vi "Dual_DM_Control_Main_V6.vi"() -> ()   [LabVIEW 2014]
uses:
  Controls/MirrorModes.ctl
  Controls/Standard Action.ctl
  <vilib>/Analysis/baseanly.llb/Mean (DBL).vi
  <vilib>/Utility/file.llb/Write To Spreadsheet File (DBL).vi
  <vilib>/Utility/file.llb/Read From Spreadsheet File (DBL).vi
  <vilib>/Analysis/NI_AALBase.lvlib
panel:
  out "Pixel Map (-1 to 1) 2":dbl[][](graph)
  in  "Python":bool
  in  "Control Mode":T1(radio)
  in  "Active Mirror":enum32{"Mirror 1", "Mirror 2"}(radio)
  in  "Clear Modes":bool
  in  "Mirror Modes":T2
  in  "Load Modes":bool
  in  "Save Modes":bool
  in  "Scan Modes":bool
  in  "Load Flat":bool
  in  "Apply Zero":bool
  in  "Load V Map":bool
  in  "Save V Map":bool
  in  "Apply Flat":bool=TRUE
  in  "Center Bias":bool
  in  "Exit":bool
  out "Pixel Map (-1 to 1)":dbl[][](graph)
  # "Mode"
  # "Amount (nm)"
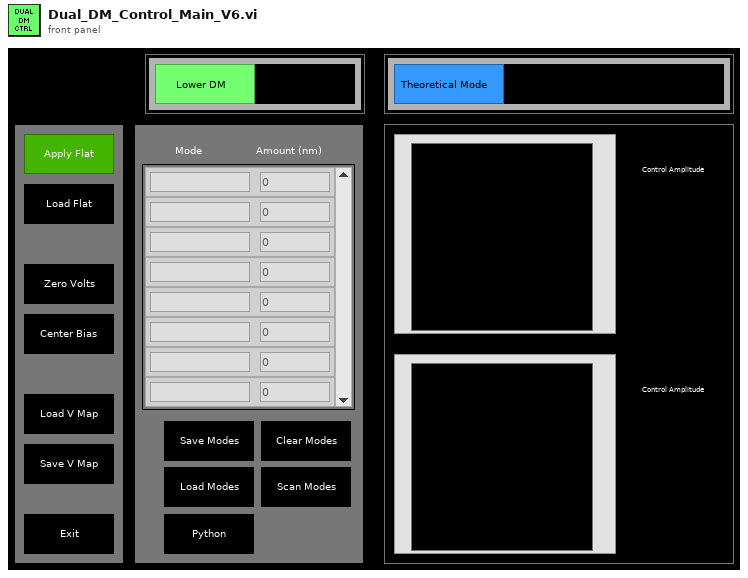
[diagram p1: front panel]
types:
  T1 = enum32{"Theoretical Mode", "Practical Mode", "Poke"}
  T2 = typedef "MirrorModes.ctl" = cluster{"Mode":string, "Amplitude":dbl}[]
  T3 = typedef "Standard Action.ctl" = enum16{"Read", "Write"}
  T4 = typedef "MirrorModes_DUAL.ctl" = cluster{"Mode":string, "Amplitude":dbl}[][]
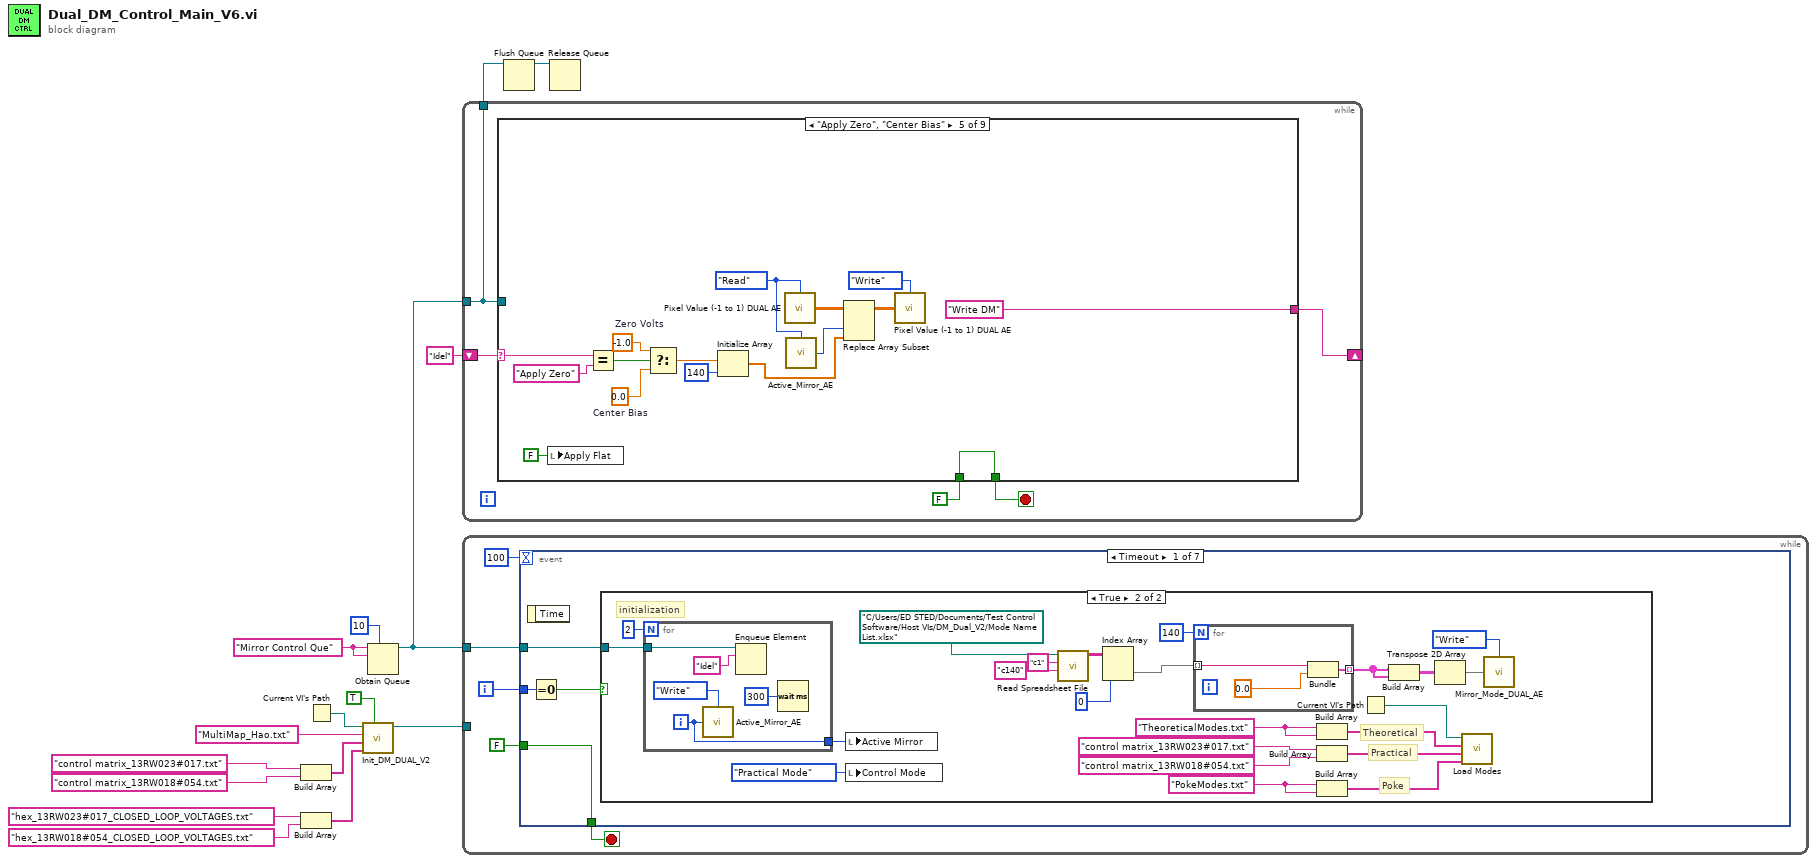
[diagram p0: block diagram]
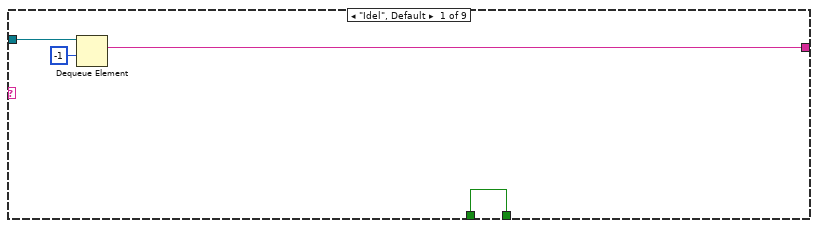
[diagram p2: hidden frame]
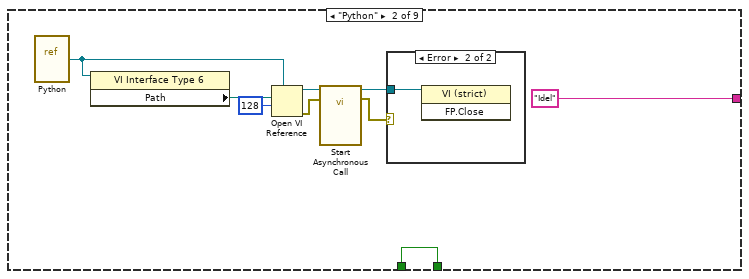
[diagram p3: hidden frame]
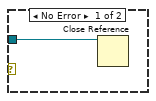
[diagram p4: hidden frame]
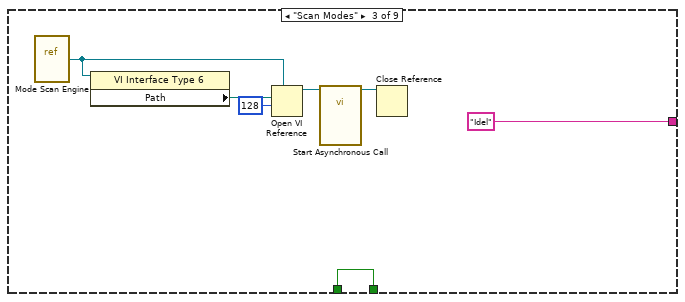
[diagram p5: hidden frame]
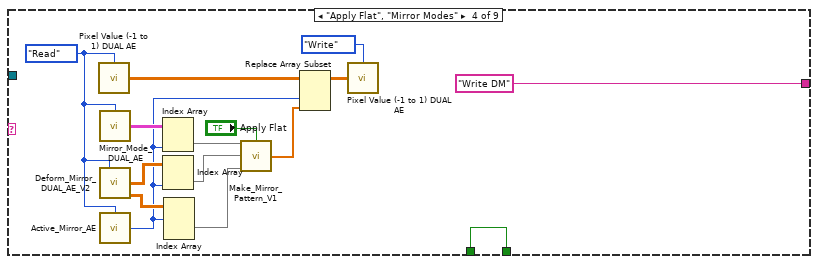
[diagram p6: hidden frame]
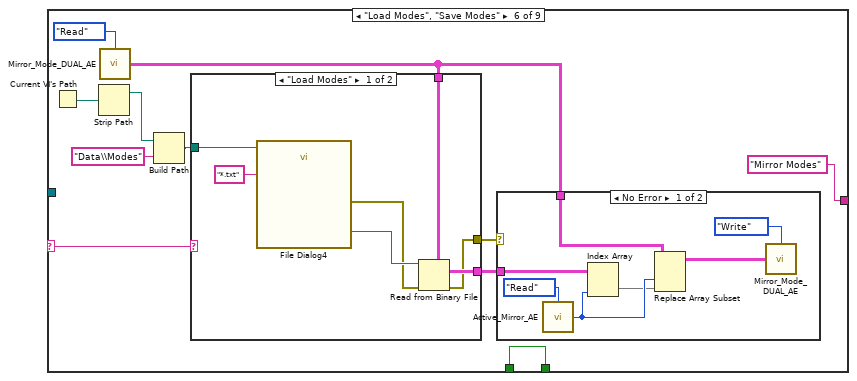
[diagram p7: hidden frame]
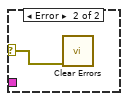
[diagram p8: hidden frame]
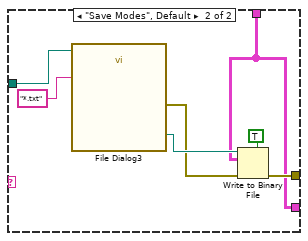
[diagram p9: hidden frame]
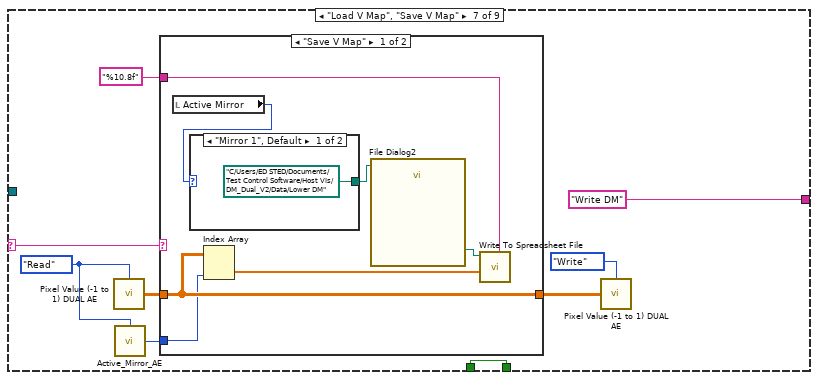
[diagram p10: hidden frame]
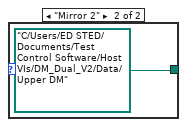
[diagram p11: hidden frame]
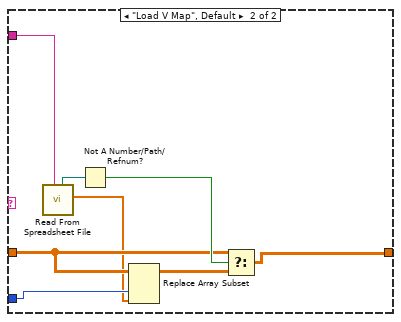
[diagram p12: hidden frame]
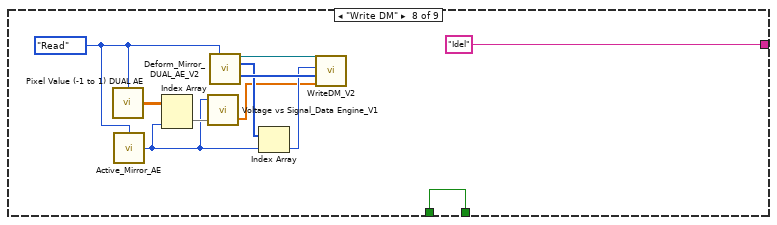
[diagram p13: hidden frame]
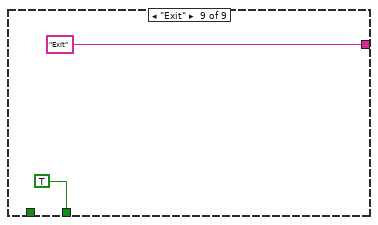
[diagram p14: hidden frame]
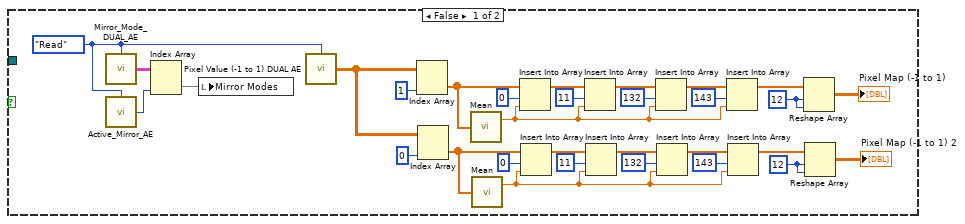
[diagram p15: hidden frame]
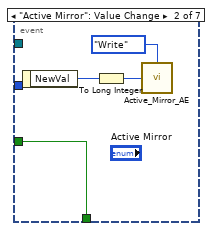
[diagram p16: hidden frame]
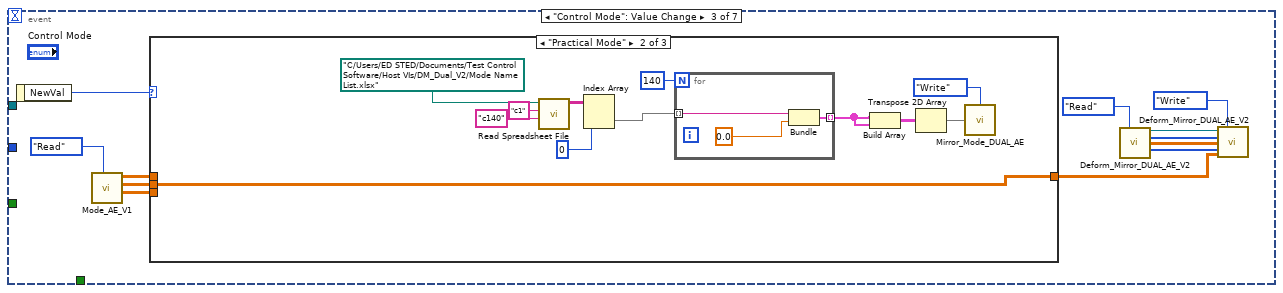
[diagram p17: hidden frame]
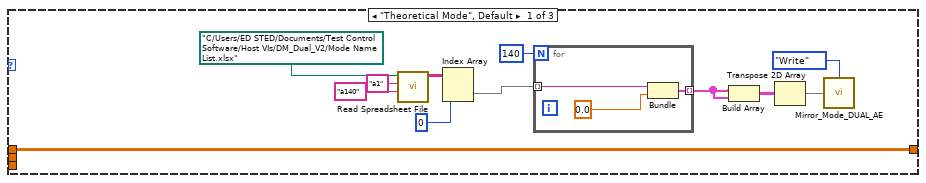
[diagram p18: hidden frame]
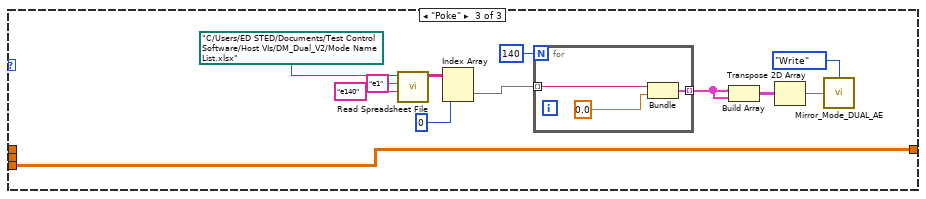
[diagram p19: hidden frame]
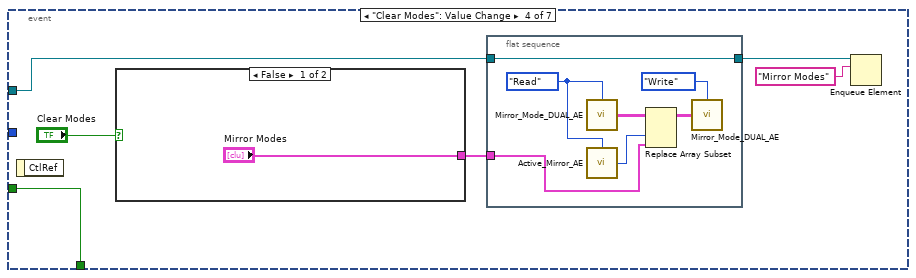
[diagram p20: hidden frame]
diagram:
  w16 = "Mirror Control Que" ("name (unnamed)")
  n1 = Build Array("control matrix_13RW023#017.txt" ("name or relative path"), "control matrix_13RW018#054.txt" ("name or relative path")) -> (w3:string[])
  n2 = Build Array("hex_13RW023#017_CLOSED_LOOP_VOLTAGES.txt" ("name or relative path"), "hex_13RW018#054_CLOSED_LOOP_VOLTAGES.txt" ("name or relative path")) -> (w6:string[])
  n3 = Current VI's Path() -> (path=w8:path)
  n4 = call "Init_DM_DUAL_V2.vi"("BM Flat"=TRUE, "BM Flat File"=w6, "Control Mode In"=w3, "DM Mapping File"="MultiMap_Hao.txt" ("name or relative path"), "Base File Path"=w8) -> ("reference out"=w14:refnum<k7>)  [unwired: 6 in]
  n5 = Obtain Queue(max queue size (-1, unlimited)=10, name (unnamed)=w16, element data type=w16) -> (queue out=w10:refnum<queue>)  [unwired: 2 in, 2 out]
  n6 = while {
    tunnel: w10 -> [w17]
    shift-right: [w21] -> _
    shift-left: "Idel" ("name (unnamed)") -> [w20]
    tunnel: [w17] -> w13
    stop <- w19 stop-if-true
    n7 = case shown="\"Apply Zero\", \"Center Bias\"" w20 {
      selector: w20 -> [_ _ _ _ w70 w82 w115 _ _]
      tunnel: w17 -> [w25 _ _ _ _ _ _ _ _]
      tunnel: [w23 "Idel" ("name (unnamed)") "Idel" ("name (unnamed)") "Write DM" ("name (unnamed)") "Write DM" ("name (unnamed)") "Mirror Modes" ("name (unnamed)") "Write DM" ("name (unnamed)") "Idel" ("name (unnamed)") "Exit" ("name (unnamed)")] -> w21
      tunnel: [w22 w28 w42 w57 w74 w85 w116 w144 TRUE] -> w19
      tunnel: FALSE -> [w22 w28 w42 w57 w74 w85 w116 w144 _]
      frame "Idel", Default {
        n8 = Dequeue Element(queue=w25, timeout in ms (-1)=-1) -> (element=w23:string)  [unwired: 1 in, 3 out]
      }
      frame "Python" {
        n9 = vi-ref "Python.vi"() -> (w29:refnum<vi>)
        n10 = property class="VI Interface Type 6"(reference=w29) -> ("Path"=w30:path)  [unwired: 1 in, 2 out]
        n11 = Open VI Reference(type specifier VI Refnum (for type only)=w29, vi path=w30, options=128) -> (vi reference=w32:refnum<vi>, error out=w27:errorcluster)  [unwired: 3 in]
        n12 = call-by-ref "Start Asynchronous Call"(reference=w32, error in=w27) -> (reference out=w33:refnum<vi>, error out=w26:errorcluster)  [unwired: 2 in]
        n13 = case shown="Error" w26 {
          tunnel: w33 -> [w35 w36]
          frame No Error {
            n14 = Close Reference(reference=w35) -> ()  [unwired: 1 in, 1 out]
          }
          frame Error {
            n15 = invoke class="VI (strict)" method="FP.Close"(reference=w36) -> ()  [unwired: 2 in, 3 out]
          }
        }
      }
      frame "Scan Modes" {
        n16 = vi-ref "Mode Scan Engine.vi"() -> (w37:refnum<vi>)
        n17 = property class="VI Interface Type 6"(reference=w37) -> ("Path"=w38:path)  [unwired: 1 in, 2 out]
        n18 = Open VI Reference(type specifier VI Refnum (for type only)=w37, vi path=w38, options=128) -> (vi reference=w40:refnum<vi>)  [unwired: 3 in, 1 out]
        n19 = call-by-ref "Start Asynchronous Call"(reference=w40) -> (reference out=w41:refnum<vi>)  [unwired: 3 in, 1 out]
        n20 = Close Reference(reference=w41) -> ()  [unwired: 1 in, 1 out]
      }
      frame "Apply Flat", "Mirror Modes" {
        w53 = Standard_Action."Read" ("Action")
        n21 = call "Pixel Value (-1 to 1) DUAL AE.vi"("Action"=w53) -> ("Pixel Value (-1 to 1) Out"=w54:dbl[][])  [unwired: 14 in]
        n22 = call "Mirror_Mode_DUAL_AE.vi"("Action"=w53) -> ("Mirror Modes Out"=w50:T4)  [unwired: 14 in]
        n23 = call "Deform_Mirror_DUAL_AE_V2.vi"("Action"=w53) -> ("Flat Files Out"=w48:dbl[][], "Mode Matrix Out"=w46:dbl[][][])  [unwired: 10 in, 3 out]
        n24 = call "Active_Mirror_AE.vi"("Action"=w53) -> ("Active Mirror"=w44:i32)  [unwired: 14 in]
        n25 = Index Array(array=w50, index (col)=w44) -> (element=w51:cluster{"Mode":string, "Amplitude":dbl}[])  [unwired: 1 in]
        n26 = Index Array(array=w48, index (col)=w44) -> (element=w49:dbl[])  [unwired: 1 in]
        n27 = Index Array(array=w46, index (dim 0)=w44) -> (element=w45:dbl[][])  [unwired: 2 in]
        n28 = call "Make_Mirror_Pattern_V1.vi"("Mirror Modes In"=w51, "Flat On?"="Apply Flat", "Flat File In"=w49, "Mirror Modes Array"=w45) -> ("Pixel Value U (-1 to 1)"=w55:dbl[])  [unwired: 11 in]
        n29 = Replace Array Subset(array=w54, new element=w55, index (col)=w44) -> (w56:dbl[][])  [unwired: 1 in]
        n30 = call "Pixel Value (-1 to 1) DUAL AE.vi"("Action"=Standard_Action."Write", "Pixel Value (-1 to 1)"=w56) -> ()  [unwired: 13 in, 1 out]
      }
      frame "Apply Zero", "Center Bias" {
        w63 = Standard_Action."Read" ("Action")
        w66 = -1.0  # Zero Volts
        w68 = 0.0  # Center Bias
        n31 = local write "Apply Flat"(FALSE ("Apply Flat")) -> ()
        n32 = Equal?(x=w70, y="Apply Zero") -> (x = y?=w69:bool)
        n33 = Select(t=w66, s=w69, f=w68) -> (s? t:f=w67:dbl)
        n34 = Initialize Array(w67, 140 ("dimension size")) -> (w60:dbl[])
        n35 = call "Pixel Value (-1 to 1) DUAL AE.vi"("Action"=w63) -> ("Pixel Value (-1 to 1) Out"=w61:dbl[][])  [unwired: 14 in]
        n36 = call "Active_Mirror_AE.vi"("Action"=w63) -> ("Active Mirror"=w62:i32)  [unwired: 14 in]
        n37 = Replace Array Subset(array=w61, new element=w60, index (col)=w62) -> (w64:dbl[][])  [unwired: 1 in]
        n38 = call "Pixel Value (-1 to 1) DUAL AE.vi"("Action"=Standard_Action."Write", "Pixel Value (-1 to 1)"=w64) -> ()  [unwired: 13 in, 1 out]
      }
      frame "Load Modes", "Save Modes" {
        n39 = Current VI's Path() -> (path=w80:path)
        n40 = Strip Path(path=w80) -> (stripped path=w79:path)  [unwired: 1 out]
        n41 = call "Mirror_Mode_DUAL_AE.vi"("Action"=Standard_Action."Read") -> ("Mirror Modes Out"=w75:T4)  [unwired: 14 in]
        n42 = Build Path(base path=w79, name or relative path="Data\\Modes") -> (appended path=w77:path)
        n43 = case shown="\"Load Modes\"" w82 {
          tunnel: w75 -> [w94 w101]
          tunnel: [w100 w101] -> w81
          tunnel: w77 -> [w99 w106]
          tunnel: [w96 w103] -> w76
          frame "Load Modes" {
            n44 = call "File Dialog4"("start path"=w99, "pattern (all files)"="*.txt") -> ("selected path"=w98:path, "error out"=w95:errorcluster)  [unwired: 10 in, 2 out]
            n45 = Read from Binary File(5:w94, 8:w95, 11:w98) -> (0:w96:errorcluster, 2:w100:T4)  [unwired: 3 in, 2 out]
          }
          frame "Save Modes", Default {
            n46 = call "File Dialog3"("start path"=w106, "pattern (all files)"="*.txt") -> ("selected path"=w105:path, "error out"=w102:errorcluster)  [unwired: 10 in, 2 out]
            n47 = Write to Binary File(file (use dialog)=w105, data=w101, error in=w102, 5:TRUE ("prepend array or string size? (T)")) -> (error out=w103:errorcluster)  [unwired: 2 in, 2 out]
          }
        }
        n48 = case shown="No Error" w76 {
          selector: w76 -> [_ w93]
          tunnel: w81 -> [w91 _]
          tunnel: w75 -> [w89 _]
          frame No Error {
            n49 = call "Active_Mirror_AE.vi"("Action"=Standard_Action."Read") -> ("Active Mirror"=w88:i32)  [unwired: 14 in]
            n50 = Index Array(array=w91, index (col)=w88) -> (element=w87:cluster{"Mode":string, "Amplitude":dbl}[])  [unwired: 1 in]
            n51 = Replace Array Subset(array=w89, new element=w87, index (col)=w88) -> (w86:T4)  [unwired: 1 in]
            n52 = call "Mirror_Mode_DUAL_AE.vi"("Action"=Standard_Action."Write", "Mirror Modes In"=w86) -> ()  [unwired: 13 in, 1 out]
          }
          frame Error {
            n53 = call <vilib>:"Clear Errors.vi"("error in (no error)"=w93) -> ()  [unwired: 5 in, 2 out]
          }
        }
      }
      frame "Load V Map", "Save V Map" {
        w109 = Standard_Action."Read" ("Action")
        n54 = call "Pixel Value (-1 to 1) DUAL AE.vi"("Action"=w109) -> ("Pixel Value (-1 to 1) Out"=w113:dbl[][])  [unwired: 14 in]
        n55 = call "Active_Mirror_AE.vi"("Action"=w109) -> ("Active Mirror"=w108:i32)  [unwired: 14 in]
        n56 = case shown="\"Save V Map\"" w115 {
          tunnel: w113 -> [w122 w129]
          tunnel: "%10.8f" -> [w123 w133]
          tunnel: [w122 w130] -> w110
          tunnel: w108 -> [w120 w128]
          frame "Save V Map" {
            n57 = local read "Active Mirror"() -> (w118:enum32{"Mirror 1", "Mirror 2"})
            n58 = case shown="\"Mirror 1\", Default" w118 {
              tunnel: [path "C:/Users/ED STED/Documents/Test Control Software/Host VIs/DM_Dual_V2/Data/Lower DM" path "C:/Users/ED STED/Documents/Test Control Software/Host VIs/DM_Dual_V2/Data/Upper DM"] -> w117
              frame "Mirror 1", Default {
              }
              frame "Mirror 2" {
              }
            }
            n59 = Index Array(array=w122, index (col)=w120) -> (element=w121:dbl[])  [unwired: 1 in]
            n60 = call "File Dialog2"("start path"=w117) -> ("selected path"=w119:path)  [unwired: 11 in, 3 out]
            n61 = call-poly <vilib>:"Write To Spreadsheet File.vi"("format (%.3f)"=w123, "1D data"=w121, "file path (dialog if empty)"=w119) -> ()  [unwired: 5 in, 1 out]
          }
          frame "Load V Map", Default {
            n62 = call-poly <vilib>:"Read From Spreadsheet File.vi"("format (%.3f)"=w133) -> ("first row"=w127:dbl[], "new file path (Not A Path if cancelled)"=w132:path)  [unwired: 6 in, 3 out]
            n63 = Not A Number/Path/Refnum?(number/path/refnum=w132) -> (NaN/Path/Refnum?=w131:bool)
            n64 = Replace Array Subset(array=w129, new element=w127, index (col)=w128) -> (w126:dbl[][])  [unwired: 1 in]
            n65 = Select(t=w129, s=w131, f=w126) -> (s? t:f=w130:dbl[][])
          }
        }
        n66 = call "Pixel Value (-1 to 1) DUAL AE.vi"("Action"=Standard_Action."Write", "Pixel Value (-1 to 1)"=w110) -> ()  [unwired: 13 in, 1 out]
      }
      frame "Write DM" {
        w139 = Standard_Action."Read" ("Action")
        n67 = call "Pixel Value (-1 to 1) DUAL AE.vi"("Action"=w139) -> ("Pixel Value (-1 to 1) Out"=w140:dbl[][])  [unwired: 14 in]
        n68 = call "Active_Mirror_AE.vi"("Action"=w139) -> ("Active Mirror"=w134:i32)  [unwired: 14 in]
        n69 = Index Array(array=w140, index (col)=w134) -> (element=w135:dbl[])  [unwired: 1 in]
        n70 = call "Voltage vs Signal_Data Engine_V1.vi"("Control Signal In (-1~1)"=w135, "DM #"=w134) -> ("Voltage Out (0~Max. Vol.)"=w136:dbl[])  [unwired: 1 in, 1 out]
        n71 = call "Deform_Mirror_DUAL_AE_V2.vi"("Action"=w139) -> ("Refnum Out"=w142:refnum<k7>, "IDs Out"=w138:i32[], "Multi Map Data Out"=w141:i32[])  [unwired: 10 in, 2 out]
        n72 = Index Array(array=w138, index=w134) -> (element=w137:i32)
        n73 = call "WriteDM_V2.vi"("reference in"=w142, "nDevId"=w137, "MultiDM  Mapping"=w141, "Voltage Array in"=w136) -> ()  [unwired: 2 in, 2 out]
      }
      frame "Exit" {
      }
    }
  }
  n74 = while {
    tunnel: w10 -> [w147]
    tunnel: w14 -> [_]
    i -> [w148]
    stop <- w151 stop-if-true
    n75 = event shown="[0] Timeout" {
      selector: _ -> [_ _ _ _ _ _ _]
      dyn-events: _ -> [_ _ _ _ _ _ _]
      timeout: 100 -> [_ _ _ _ _ _ _]
      tunnel: [w155 w221 _ w284 w304 w309 w346] -> w151
      tunnel: FALSE -> [w155 w221 _ w284 w304 w309 _]
      tunnel: w148 -> [w154 _ _ _ _ _ _]
      tunnel: w147 -> [w152 _ _ w283 w303 _ w344]
      event Timeout {
        n76 = event-data() -> ()  [unwired: 1 in, 1 out]
        n77 = Equal To 0?(x=w154) -> (x = 0?=w153:bool)
        n78 = case shown="True" w153 {
          tunnel: w152 -> [_ w209]
          frame False {
            w159 = 12 ("dimension size")
            w183 = 12 ("dimension size")
            w184 = Standard_Action."Read" ("Action")
            n79 = call "Mirror_Mode_DUAL_AE.vi"("Action"=w184) -> ("Mirror Modes Out"=w171:T4)  [unwired: 14 in]
            n80 = call "Active_Mirror_AE.vi"("Action"=w184) -> ("Active Mirror"=w185:i32)  [unwired: 14 in]
            n81 = Index Array(array=w171, index (col)=w185) -> (element=w172:cluster{"Mode":string, "Amplitude":dbl}[])  [unwired: 1 in]
            n82 = local write "Mirror Modes"(w172) -> ()
            n83 = call "Pixel Value (-1 to 1) DUAL AE.vi"("Action"=w184) -> ("Pixel Value (-1 to 1) Out"=w157:dbl[][])  [unwired: 14 in]
            n84 = Index Array(array=w157, index (col)=1 ("disabled index (col)")) -> (element=w186:dbl[])  [unwired: 1 in]
            n85 = Index Array(array=w157, index (col)=0 ("disabled index (col)")) -> (element=w158:dbl[])  [unwired: 1 in]
            n86 = call-poly <vilib>:"Mean.vi"("X"=w186) -> ("mean"=w181:dbl)  [unwired: 1 out]
            n87 = call-poly <vilib>:"Mean.vi"("X"=w158) -> ("mean"=w160:dbl)  [unwired: 1 out]
            n88 = Insert Into Array(array=w186, index=0, new element=w181) -> (w176:dbl[])
            n89 = Insert Into Array(array=w158, index=0, new element=w160) -> (w165:dbl[])
            n90 = Insert Into Array(array=w176, index=11, new element=w181) -> (w178:dbl[])
            n91 = Insert Into Array(array=w165, index=11, new element=w160) -> (w163:dbl[])
            n92 = Insert Into Array(array=w178, index=132, new element=w181) -> (w180:dbl[])
            n93 = Insert Into Array(array=w163, index=132, new element=w160) -> (w161:dbl[])
            n94 = Insert Into Array(array=w180, index=143, new element=w181) -> (w173:dbl[])
            n95 = Insert Into Array(array=w161, index=143, new element=w160) -> (w168:dbl[])
            n96 = Reshape Array(w173, w183, w183) -> (→"Pixel Map (-1 to 1)":dbl[][])
            n97 = Reshape Array(w168, w159, w159) -> (→"Pixel Map (-1 to 1) 2":dbl[][])
          }
          frame True {
            w192 = "PokeModes.txt" ("name or relative path")
            w189 = "TheoreticalModes.txt" ("name or relative path")
            # "initialization"
            # "Poke"
            # "Practical"
            # "Theoretical"
            n98 = for {
              N: 2 -> [_]
              tunnel: w209 -> [w214]
              tunnel: [w210] -> w203
              i -> [w210]
              n99 = call "Active_Mirror_AE.vi"("Action"=Standard_Action."Write", "Active Mirror In"=w210) -> ()  [unwired: 13 in, 1 out]
              n100 = Enqueue Element(queue=w214, element="Idel") -> ()  [unwired: 2 in, 3 out]
              n101 = Wait (ms)(milliseconds to wait=u32 300) -> ()  [unwired: 1 out]
            }
            n102 = local write "Active Mirror"(w203) -> ()
            n103 = local write "Control Mode"(T1."Practical Mode" ("Control Mode")) -> ()
            n104 = call "Read Spreadsheet File.vi"("End cell"="c140", "Start Cell"="c1", "path"=path "C:/Users/ED STED/Documents/Test Control Software/Host VIs/DM_Dual_V2/Mode Name List.xlsx") -> ("Array"=w198:string[][])  [unwired: 7 in, 1 out]
            n105 = Index Array(array=w198, index (col)=0 ("disabled index (col)")) -> (element=w196:string[])  [unwired: 1 in]
            n106 = for {
              N: 140 -> [_]
              tunnel: [w216] -> w206 mode=indexing
              tunnel: w196 -> [w215] mode=indexing
              n107 = Bundle(w215, 0.0) -> (w216:cluster{string, dbl})  [unwired: 1 in]
            }
            n108 = Build Array(w189, w189) -> (w194:string[])
            n109 = Build Array("control matrix_13RW023#017.txt" ("name or relative path"), "control matrix_13RW018#054.txt" ("name or relative path")) -> (w193:string[])
            n110 = Build Array(w192, w192) -> (w191:string[])
            n111 = Current VI's Path() -> (path=w195:path)
            n112 = Build Array(w206, w206) -> (w204:cluster{string, dbl}[][])
            n113 = Transpose 2D Array(2D array=w204) -> (transposed array=w199:cluster{string, dbl}[][])
            n114 = call "Load Modes.vi"("Poke Path"=w191, "Practical Mode Path"=w193, "Theoretical Mode Path"=w194, "Base File Path"=w195) -> ()  [unwired: 2 in]
            n115 = call "Mirror_Mode_DUAL_AE.vi"("Action"=Standard_Action."Write", "Mirror Modes In"=w199) -> ()  [unwired: 13 in, 1 out]
          }
        }
      }
      event "Active Mirror": Value Change {
        n116 = event-data() -> ("NewVal"=w220:enum32{"Mirror 1", "Mirror 2"})  [unwired: 1 in]
        n117 = To Long Integer(number=w220) -> (32bit integer=w219:i32)
        n118 = call "Active_Mirror_AE.vi"("Action"=Standard_Action."Write", "Active Mirror In"=w219) -> ()  [unwired: 13 in, 1 out]
      }
      event "Control Mode": Value Change {
        n119 = event-data() -> ("NewVal"=w233:T1)  [unwired: 1 in]
        n120 = call "Mode_AE_V1.vi"("Action"=Standard_Action."Read") -> ("Poke Mode Out"=w228:dbl[][][], "Practical Mode Out"=w229:dbl[][][], "Theoretical Mode Out"=w230:dbl[][][])  [unwired: 7 in]
        n121 = case shown="\"Practical Mode\"" w233 {
          tunnel: w230 -> [w245 _ _]
          tunnel: w229 -> [_ w260 _]
          tunnel: w228 -> [_ _ w264]
          tunnel: [w245 w260 w264] -> w227
          frame "Theoretical Mode", Default {
            n122 = call "Read Spreadsheet File.vi"("End cell"="a140", "Start Cell"="a1", "path"=path "C:/Users/ED STED/Documents/Test Control Software/Host VIs/DM_Dual_V2/Mode Name List.xlsx") -> ("Array"=w236:string[][])  [unwired: 7 in, 1 out]
            n123 = Index Array(array=w236, index (col)=0 ("disabled index (col)")) -> (element=w234:string[])  [unwired: 1 in]
            n124 = for {
              N: 140 -> [_]
              tunnel: [w247] -> w242 mode=indexing
              tunnel: w234 -> [w246] mode=indexing
              n125 = Bundle(w246, 0.0) -> (w247:cluster{string, dbl})  [unwired: 1 in]
            }
            n126 = Build Array(w242, w242) -> (w241:cluster{string, dbl}[][])
            n127 = Transpose 2D Array(2D array=w241) -> (transposed array=w237:cluster{string, dbl}[][])
            n128 = call "Mirror_Mode_DUAL_AE.vi"("Action"=Standard_Action."Write", "Mirror Modes In"=w237) -> ()  [unwired: 13 in, 1 out]
          }
          frame "Practical Mode" {
            n129 = call "Read Spreadsheet File.vi"("End cell"="c140", "Start Cell"="c1", "path"=path "C:/Users/ED STED/Documents/Test Control Software/Host VIs/DM_Dual_V2/Mode Name List.xlsx") -> ("Array"=w251:string[][])  [unwired: 7 in, 1 out]
            n130 = Index Array(array=w251, index (col)=0 ("disabled index (col)")) -> (element=w249:string[])  [unwired: 1 in]
            n131 = for {
              N: 140 -> [_]
              tunnel: [w262] -> w257 mode=indexing
              tunnel: w249 -> [w261] mode=indexing
              n132 = Bundle(w261, 0.0) -> (w262:cluster{string, dbl})  [unwired: 1 in]
            }
            n133 = Build Array(w257, w257) -> (w256:cluster{string, dbl}[][])
            n134 = Transpose 2D Array(2D array=w256) -> (transposed array=w252:cluster{string, dbl}[][])
            n135 = call "Mirror_Mode_DUAL_AE.vi"("Action"=Standard_Action."Write", "Mirror Modes In"=w252) -> ()  [unwired: 13 in, 1 out]
          }
          frame "Poke" {
            n136 = call "Read Spreadsheet File.vi"("End cell"="e140", "Start Cell"="e1", "path"=path "C:/Users/ED STED/Documents/Test Control Software/Host VIs/DM_Dual_V2/Mode Name List.xlsx") -> ("Array"=w267:string[][])  [unwired: 7 in, 1 out]
            n137 = Index Array(array=w267, index (col)=0 ("disabled index (col)")) -> (element=w265:string[])  [unwired: 1 in]
            n138 = for {
              N: 140 -> [_]
              tunnel: [w277] -> w273 mode=indexing
              tunnel: w265 -> [w276] mode=indexing
              n139 = Bundle(w276, 0.0) -> (w277:cluster{string, dbl})  [unwired: 1 in]
            }
            n140 = Build Array(w273, w273) -> (w272:cluster{string, dbl}[][])
            n141 = Transpose 2D Array(2D array=w272) -> (transposed array=w268:cluster{string, dbl}[][])
            n142 = call "Mirror_Mode_DUAL_AE.vi"("Action"=Standard_Action."Write", "Mirror Modes In"=w268) -> ()  [unwired: 13 in, 1 out]
          }
        }
        n143 = call "Deform_Mirror_DUAL_AE_V2.vi"("Action"=Standard_Action."Read") -> ("Refnum Out"=w226:refnum<k7>, "IDs Out"=w225:i32[], "Flat Files Out"=w224:dbl[][], "Multi Map Data Out"=w223:i32[])  [unwired: 10 in, 1 out]
        n144 = call "Deform_Mirror_DUAL_AE_V2.vi"("Refnum In"=w226, "Action"=Standard_Action."Write", "IDs In"=w225, "Flat Files In"=w224, "Multi Map Data In"=w223, "Mode Matrix In"=w227) -> ()  [unwired: 5 in, 5 out]
      }
      event "Clear Modes": Value Change {
        n145 = event-data() -> ()  [unwired: 1 in, 1 out]
        n146 = case shown="False" "Clear Modes" {
          tunnel: ["Mirror Modes" w286] -> w279
          frame False {
          }
          frame True {
            w289 = Standard_Action."Read" ("Action")
            n147 = call "Mirror_Mode_DUAL_AE.vi"("Action"=w289) -> ("Mirror Modes Out"=w288:T4)  [unwired: 14 in]
            n148 = call "Active_Mirror_AE.vi"("Action"=w289) -> ("Active Mirror"=w290:i32)  [unwired: 14 in]
            n149 = Index Array(array=w288, index (col)=w290) -> (element=w287:cluster{"Mode":string, "Amplitude":dbl}[])  [unwired: 1 in]
            n150 = for {
              tunnel: w287 -> [w293] mode=indexing
              tunnel: [w291] -> w286 mode=indexing
              n151 = Bundle By Name(cluster=w293, "Amplitude"=0.0) -> (w291:cluster{"Mode":string, "Amplitude":dbl})
            }
          }
        }
        n152 = flat-sequence {
          tunnel: w279 -> [w294]
          tunnel: w283 -> [w300]
          tunnel: [w300] -> w281
          frame #0 {
            w297 = Standard_Action."Read" ("Action")
            n153 = call "Mirror_Mode_DUAL_AE.vi"("Action"=w297) -> ("Mirror Modes Out"=w296:T4)  [unwired: 14 in]
            n154 = call "Active_Mirror_AE.vi"("Action"=w297) -> ("Active Mirror"=w298:i32)  [unwired: 14 in]
            n155 = Replace Array Subset(array=w296, new element=w294, index (col)=w298) -> (w299:T4)  [unwired: 1 in]
            n156 = call "Mirror_Mode_DUAL_AE.vi"("Action"=Standard_Action."Write", "Mirror Modes In"=w299) -> ()  [unwired: 13 in, 1 out]
          }
        }
        n157 = Enqueue Element(queue=w281, element="Mirror Modes") -> ()  [unwired: 2 in, 3 out]
      }
      event "Apply Flat", "Center Bias", "Apply Zero", "Save V Map", "Save Modes", "Load Modes", "Load V Map", "Scan Modes", "Python": Value Change {
        n158 = event-data() -> ("CtlRef"=w302:refnum<vi>)  [unwired: 1 in]
        n159 = property class="Bool"(reference=w302) -> ("Label.Text"=w301:string)  [unwired: 1 in, 2 out]
        n160 = Enqueue Element(queue=w303, element=w301) -> ()  [unwired: 2 in, 3 out]
      }
      event "Load Flat": Value Change {
        n161 = event-data() -> ()  [unwired: 1 in, 1 out]
        n162 = local read "Active Mirror"() -> (w307:enum32{"Mirror 1", "Mirror 2"})
        n163 = case shown="\"Mirror 1\", Default" w307 {
          tunnel: [path "C:/Users/ED STED/Documents/Test Control Software/Host VIs/DM_Dual_V2/Data/Lower DM" path "C:/Users/ED STED/Documents/Test Control Software/Host VIs/DM_Dual_V2/Data/Upper DM"] -> w306
          frame "Mirror 1", Default {
          }
          frame "Mirror 2" {
          }
        }
        n164 = call "File Dialog"("start path"=w306) -> ("selected path"=w308:path, "error out"=w305:errorcluster)  [unwired: 11 in, 2 out]
        n165 = case shown="No Error" w305 {
          tunnel: w308 -> [w310 _]
          frame No Error {
            n166 = call-poly <vilib>:"Read From Spreadsheet File.vi"("format (%.3f)"="%10.8f", "file path (dialog if empty)"=w310) -> ("first row"=w312:dbl[], "new file path (Not A Path if cancelled)"=w314:path)  [unwired: 5 in, 3 out]
            n167 = Not A Number/Path/Refnum?(number/path/refnum=w314) -> (NaN/Path/Refnum?=w313:bool)
            n168 = case shown="False" w313 {
              tunnel: w312 -> [w331 _]
              tunnel: "Load Flat" -> [_ _]
              frame False {
                w322 = Standard_Action."Read" ("Action")
                n169 = In Range and Coerce(upper limit=1.0, x=w331, lower limit=-1.0) -> (coerced(x)=w316:dbl[], In Range?=w328:bool[])
                n170 = Not(x=w328) -> (.not. x?=w327:bool[])
                n171 = call "Deform_Mirror_DUAL_AE_V2.vi"("Action"=w322) -> ("Refnum Out"=w317:refnum<k7>, "IDs Out"=w318:i32[], "Flat Files Out"=w323:dbl[][], "Multi Map Data Out"=w319:i32[], "Mode Matrix Out"=w320:dbl[][][])  [unwired: 10 in]
                n172 = call "Active_Mirror_AE.vi"("Action"=w322) -> ("Active Mirror"=w325:i32)  [unwired: 14 in]
                n173 = Or Array Elements(Boolean array=w327) -> (logical OR=w326:bool)
                n174 = Replace Array Subset(array=w323, new element=w316, index (col)=w325) -> (w324:dbl[][])  [unwired: 1 in]
                n175 = call "Deform_Mirror_DUAL_AE_V2.vi"("Refnum In"=w317, "Action"=Standard_Action."Write", "IDs In"=w318, "Flat Files In"=w324, "Multi Map Data In"=w319, "Mode Matrix In"=w320) -> ()  [unwired: 5 in, 5 out]
                n176 = case shown="True" w326 {
                  frame False {
                  }
                  frame True {
                    n177 = One Button Dialog(message="Flat File Out of Range [-1, 1]") -> ()  [unwired: 1 in, 1 out]
                  }
                }
              }
              frame True {
              }
            }
          }
          frame Error {
          }
        }
      }
      event "Exit": Value Change {
        n178 = event-data() -> ("NewVal"=w346:bool)  [unwired: 1 in]
        n179 = for {
          N: 2 -> [_]
          tunnel: w344 -> [w352]
          tunnel: [w347] -> w335
          i -> [w348]
          n180 = call "Active_Mirror_AE.vi"("Action"=Standard_Action."Write", "Active Mirror In"=w348) -> ()  [unwired: 13 in, 1 out]
          n181 = Enqueue Element(queue=w352, element="Apply Zero") -> (queue out=w347:refnum<queue>)  [unwired: 2 in, 2 out]
          n182 = Wait (ms)(milliseconds to wait=u32 300) -> ()  [unwired: 1 out]
        }
        n183 = Enqueue Element(queue=w335, element="Exit") -> (error out=w339:errorcluster)  [unwired: 2 in, 2 out]
        n184 = call "Deform_Mirror_DUAL_AE_V2.vi"("Action"=Standard_Action."Read") -> ("Refnum Out"=w342:refnum<k7>, "IDs Out"=w337:i32[])  [unwired: 10 in, 3 out]
        n185 = call "ConfigDM.vi"("High Voltage"=FALSE, "error in (no error)"=w339, "Dev IDs"=w337, "Automation Refnum in"=w342) -> ("error out"=w338:errorcluster, "Automation Refnum out"=w341:refnum<k7>)  [unwired: 6 in]
        n186 = Close Reference(reference=w341, error in (no error)=w338) -> ()  [unwired: 1 out]
      }
    }
  }
  n187 = Flush Queue(queue=w13) -> (queue out=w12:refnum<queue>)  [unwired: 1 in, 2 out]
  n188 = Release Queue(queue=w12) -> ()  [unwired: 2 in, 3 out]
